vi "数字量输出配置.vi"() -> ()   [LabVIEW 2010] (continued)
            n7296 = local write "输入值_26"(w975) -> ()
            n7297 = local write "输入值_27"(w975) -> ()
            n7298 = local write "输入值_28"(w975) -> ()
            n7299 = local write "输入值_29"(w975) -> ()
            n7300 = local write "输入值_30"(w975) -> ()
            n7301 = local write "输入值_31"(w975) -> ()
            n7302 = local write "输入值_32"(w975) -> ()
            n7303 = local write "输入值_33"(w975) -> ()
            n7304 = local write "输入值_34"(w975) -> ()
            n7305 = local write "输入值_35"(w975) -> ()
            n7306 = local write "输入值_36"(w975) -> ()
            n7307 = local write "输入值_37"(w975) -> ()
            n7308 = local write "输入值_38"(w975) -> ()
            n7309 = local write "输入值_39"(w975) -> ()
            n7310 = local write "输入值_40"(w975) -> ()
            n7311 = local write "输入值_41"(w975) -> ()
            n7312 = local write "输入值_42"(w975) -> ()
            n7313 = local write "输入值_43"(w975) -> ()
            n7314 = local write "输入值_44"(w975) -> ()
            n7315 = local write "输入值_45"(w975) -> ()
            n7316 = local write "输入值_46"(w975) -> ()
            n7317 = local write "输入值_47"(w975) -> ()
            n7318 = local write "输入值_48"(w975) -> ()
            n7319 = local write "输入值_49"(w975) -> ()
            n7320 = local write "输入值_50"(w975) -> ()
            n7321 = local write "输入值_51"(w975) -> ()
            n7322 = local write "输入值_52"(w975) -> ()
            n7323 = local write "输入值_53"(w975) -> ()
            n7324 = local write "输入值_54"(w975) -> ()
            n7325 = local write "输入值_55"(w975) -> ()
            n7326 = local write "输入值_56"(w975) -> ()
            n7327 = local write "输入值_57"(w975) -> ()
            n7328 = local write "输入值_58"(w975) -> ()
            n7329 = local write "输入值_59"(w975) -> ()
            n7330 = local write "输入值_60"(w975) -> ()
            n7331 = local write "输入值_61"(w975) -> ()
            n7332 = local write "输入值_62"(w975) -> ()
            n7333 = local write "输入值_63"(w975) -> ()
            n7334 = local write "输入值_64"(w975) -> ()
            n7335 = local write "输入值_65"(w975) -> ()
            n7336 = local write "输入值_66"(w975) -> ()
            n7337 = local write "输入值_67"(w975) -> ()
            n7338 = local write "输入值_68"(w975) -> ()
            n7339 = local write "输入值_69"(w975) -> ()
            n7340 = local write "输入值_70"(w975) -> ()
            n7341 = local write "输入值_71"(w975) -> ()
            n7342 = local write "输入值_72"(w975) -> ()
            n7343 = local write "输入值_73"(w975) -> ()
            n7344 = local write "输入值_74"(w975) -> ()
            n7345 = local write "输入值_75"(w975) -> ()
            n7346 = local write "输入值_76"(w975) -> ()
            n7347 = local write "输入值_77"(w975) -> ()
            n7348 = local write "输入值_78"(w975) -> ()
            n7349 = local write "输入值_79"(w975) -> ()
            n7350 = local write "输入值_80"(w975) -> ()
          }
          event "btn_置0": Value Change {
            w976 = enum16{"0", "1"}."0" ("输入值_41")
            n7351 = event-data() -> ()  [unwired: 1 in, 5 out]
            n7352 = local write "输入值_1"(w976) -> ()
            n7353 = local write "输入值_2"(w976) -> ()
            n7354 = local write "输入值_3"(w976) -> ()
            n7355 = local write "输入值_4"(w976) -> ()
            n7356 = local write "输入值_5"(w976) -> ()
            n7357 = local write "输入值_6"(w976) -> ()
            n7358 = local write "输入值_7"(w976) -> ()
            n7359 = local write "输入值_8"(w976) -> ()
            n7360 = local write "输入值_9"(w976) -> ()
            n7361 = local write "输入值_10"(w976) -> ()
            n7362 = local write "输入值_11"(w976) -> ()
            n7363 = local write "输入值_12"(w976) -> ()
            n7364 = local write "输入值_13"(w976) -> ()
            n7365 = local write "输入值_14"(w976) -> ()
            n7366 = local write "输入值_15"(w976) -> ()
            n7367 = local write "输入值_16"(w976) -> ()
            n7368 = local write "输入值_17"(w976) -> ()
            n7369 = local write "输入值_18"(w976) -> ()
            n7370 = local write "输入值_19"(w976) -> ()
            n7371 = local write "输入值_20"(w976) -> ()
            n7372 = local write "输入值_21"(w976) -> ()
            n7373 = local write "输入值_22"(w976) -> ()
            n7374 = local write "输入值_23"(w976) -> ()
            n7375 = local write "输入值_24"(w976) -> ()
            n7376 = local write "输入值_25"(w976) -> ()
            n7377 = local write "输入值_26"(w976) -> ()
            n7378 = local write "输入值_27"(w976) -> ()
            n7379 = local write "输入值_28"(w976) -> ()
            n7380 = local write "输入值_29"(w976) -> ()
            n7381 = local write "输入值_30"(w976) -> ()
            n7382 = local write "输入值_31"(w976) -> ()
            n7383 = local write "输入值_32"(w976) -> ()
            n7384 = local write "输入值_33"(w976) -> ()
            n7385 = local write "输入值_34"(w976) -> ()
            n7386 = local write "输入值_35"(w976) -> ()
            n7387 = local write "输入值_36"(w976) -> ()
            n7388 = local write "输入值_37"(w976) -> ()
            n7389 = local write "输入值_38"(w976) -> ()
            n7390 = local write "输入值_39"(w976) -> ()
            n7391 = local write "输入值_40"(w976) -> ()
            n7392 = local write "输入值_41"(w976) -> ()
            n7393 = local write "输入值_42"(w976) -> ()
            n7394 = local write "输入值_43"(w976) -> ()
            n7395 = local write "输入值_44"(w976) -> ()
            n7396 = local write "输入值_45"(w976) -> ()
            n7397 = local write "输入值_46"(w976) -> ()
            n7398 = local write "输入值_47"(w976) -> ()
            n7399 = local write "输入值_48"(w976) -> ()
            n7400 = local write "输入值_49"(w976) -> ()
            n7401 = local write "输入值_50"(w976) -> ()
            n7402 = local write "输入值_51"(w976) -> ()
            n7403 = local write "输入值_52"(w976) -> ()
            n7404 = local write "输入值_53"(w976) -> ()
            n7405 = local write "输入值_54"(w976) -> ()
            n7406 = local write "输入值_55"(w976) -> ()
            n7407 = local write "输入值_56"(w976) -> ()
            n7408 = local write "输入值_57"(w976) -> ()
            n7409 = local write "输入值_58"(w976) -> ()
            n7410 = local write "输入值_59"(w976) -> ()
            n7411 = local write "输入值_60"(w976) -> ()
            n7412 = local write "输入值_61"(w976) -> ()
            n7413 = local write "输入值_62"(w976) -> ()
            n7414 = local write "输入值_63"(w976) -> ()
            n7415 = local write "输入值_64"(w976) -> ()
            n7416 = local write "输入值_65"(w976) -> ()
            n7417 = local write "输入值_66"(w976) -> ()
            n7418 = local write "输入值_67"(w976) -> ()
            n7419 = local write "输入值_68"(w976) -> ()
            n7420 = local write "输入值_69"(w976) -> ()
            n7421 = local write "输入值_70"(w976) -> ()
            n7422 = local write "输入值_71"(w976) -> ()
            n7423 = local write "输入值_72"(w976) -> ()
            n7424 = local write "输入值_73"(w976) -> ()
            n7425 = local write "输入值_74"(w976) -> ()
            n7426 = local write "输入值_75"(w976) -> ()
            n7427 = local write "输入值_76"(w976) -> ()
            n7428 = local write "输入值_77"(w976) -> ()
            n7429 = local write "输入值_78"(w976) -> ()
            n7430 = local write "输入值_79"(w976) -> ()
            n7431 = local write "输入值_80"(w976) -> ()
          }
        }
      }
      n7432 = Obtain Notifier(name (unnamed)=w188, notification data type=w188) -> (notifier out=w190:refnum<notifier>, error out=w189:errorcluster)  [unwired: 2 in, 1 out]
      n7433 = while {
        tunnel: w190 -> [w477]
        tunnel: w189 -> [w476]
        tunnel: [w475] -> w187
        tunnel: [w474] -> w186
        stop <- w478 stop-if-true
        n7434 = Wait Until Next ms Multiple(millisecond multiple=u32 20 ("毫秒倍数")) -> ()  [unwired: 1 out]
        n7435 = Wait on Notification(notifier=w477, timeout in ms (-1)=20 ("超时毫秒(-1)"), error in (no error)=w476) -> (notifier out=w475:refnum<notifier>, notification=w483:string, error out=w474:errorcluster)  [unwired: 1 in, 1 out]
        n7436 = Equal?(x=w483, y="DOutput" ("通知")) -> (x = y?=w481:bool)
        n7437 = case shown="真" w481 {
          frame False {
          }
          frame True {
            n7438 = while {
              stop <- w485 stop-if-true
              n7439 = local read "保持输出"() -> (w484:bool)
              n7440 = case shown="真" w484 {
                selector: w484 -> [_ w519]
                tunnel: [w490 w520] -> w487
                tunnel: [w489 w518] -> w486
                frame False {
                  n7441 = stacked-sequence {
                    tunnel: [_ w514] -> w489
                    tunnel: [w492 _] -> w490
                    frame #0 {
                      n7442 = local read "同步_A2"() -> (w494:i32)
                      n7443 = local read "同步_A1"() -> (w491:i32)
                      n7444 = Equal?(x=w491, y=w494) -> (x = y?=w493:bool)
                      n7445 = case shown="真" w493 {
                        tunnel: [FALSE w496] -> w492
                        frame False {
                        }
                        frame True {
                          n7446 = stacked-sequence {
                            tunnel: [_ w506 _] -> w496
                            frame #0 {
                              w498 = "DOCheckStart" ("名称（未命名）")
                              n7447 = Obtain Notifier(name (unnamed)=w498, notification data type=w498) -> (notifier out=w499:refnum<notifier>)  [unwired: 2 in, 2 out]
                              n7448 = Send Notification(notification="DOCheck" ("通知"), notifier=w499) -> ()  [unwired: 1 in, 2 out]
                            }
                            frame #1 {
                              # "32+16+PWM+16(I/O)\n4X3=12   每次一组"
                              # "以太网发送修改数字量输出参数命令"
                              n7449 = local read "数组_输入值"() -> (w508:enum16{"0", "1"}[][])
                              n7450 = local read "同步_A1"() -> (w504:i32)
                              n7451 = call "数值转换为U16.vi"("数值数组输入"=w508) -> ("U16输出"=w505:u16[])  [unwired: 10 in]
                              n7452 = Multiply(x=w504, y=3) -> (x*y=w502:i32)
                              n7453 = Array Subset(array=w505, index=w502, length=3 ("长度")) -> (w500:u16[])
                              n7454 = call "UDP发送.vi"("发送数据"=w500, "数据区字长"=u16 3, "报文类型"=u16 1285, "发送方标识"=u16 5397) -> ("Error"=w507:cluster{"错误？":bool, "数值":i32, "字符串":string})  [unwired: 6 in]
                              n7455 = Unbundle By Name(w507) -> ("错误？"=w506:bool)
                            }
                            frame #2 {
                              n7456 = local read "同步_A1"() -> (w512:i32)
                              n7457 = Increment(x=w512) -> (x+1=w513:i32)
                              n7458 = local write "同步_A1"(w513) -> ()
                            }
                          }
                        }
                      }
                    }
                    frame #1 {
                      n7459 = local read "同步_A1"() -> (w515:i32)
                      n7460 = Equal?(x=w515, y=5) -> (x = y?=w514:bool)
                      n7461 = case shown="真" w514 {
                        frame False {
                        }
                        frame True {
                          n7462 = property on="保持输出" class="Bool (严格)"("DisabledEnum"=T1."Enabled" ("禁用")) -> ()  [unwired: 2 in, 2 out]
                        }
                      }
                    }
                  }
                }
                frame True {
                  n7463 = Not(x=w519) -> (.not. x?=w518:bool)
                  n7464 = stacked-sequence {
                    tunnel: [_ w530] -> w520
                    frame #0 {
                      w522 = "DOCheckStart" ("名称（未命名）")
                      n7465 = Obtain Notifier(name (unnamed)=w522, notification data type=w522) -> (notifier out=w523:refnum<notifier>)  [unwired: 2 in, 2 out]
                      n7466 = Send Notification(notification="DOCheck" ("通知"), notifier=w523) -> ()  [unwired: 1 in, 2 out]
                    }
                    frame #1 {
                      # "32+16+PWM+16(I/O)\n4X3=12，每次一组"
                      # "以太网发送修改数字量输出参数命令"
                      n7467 = local read "数组_输入值"() -> (w532:enum16{"0", "1"}[][])
                      n7468 = local read "同步_A1"() -> (w528:i32)
                      n7469 = call "数值转换为U16.vi"("数值数组输入"=w532) -> ("U16输出"=w529:u16[])  [unwired: 10 in]
                      n7470 = Multiply(x=w528, y=3) -> (x*y=w526:i32)
                      n7471 = Array Subset(array=w529, index=w526, length=3 ("长度")) -> (w524:u16[])
                      n7472 = call "UDP发送.vi"("发送数据"=w524, "数据区字长"=u16 3, "报文类型"=u16 1285, "发送方标识"=u16 5397) -> ("Error"=w531:cluster{"错误？":bool, "数值":i32, "字符串":string})  [unwired: 6 in]
                      n7473 = Unbundle By Name(w531) -> ("错误？"=w530:bool)
                    }
                  }
                }
              }
              n7474 = Wait Until Next ms Multiple(millisecond multiple=u32 25 ("毫秒倍数")) -> ()  [unwired: 1 out]
              n7475 = Or(x=w487, y=w486) -> (x .or. y?=w485:bool)
            }
          }
        }
        n7476 = local read "关闭？"() -> (w478:bool)
      }
      n7477 = Release Notifier(notifier=w187, error in (no error)=w186) -> ()  [unwired: 1 in, 3 out]
      n7478 = Obtain Notifier(name (unnamed)=w185, notification data type=w185) -> (notifier out=w184:refnum<notifier>, error out=w183:errorcluster)  [unwired: 2 in, 1 out]
      n7479 = while {
        tunnel: w184 -> [w194]
        tunnel: w183 -> [w193]
        tunnel: [w192] -> w182
        tunnel: [w191] -> w181
        stop <- w196 stop-if-true
        n7480 = Wait Until Next ms Multiple(millisecond multiple=u32 20 ("毫秒倍数")) -> ()  [unwired: 1 out]
        n7481 = Wait on Notification(notifier=w194, timeout in ms (-1)=20 ("超时毫秒(-1)"), error in (no error)=w193) -> (notifier out=w192:refnum<notifier>, notification=w197:string, error out=w191:errorcluster)  [unwired: 1 in, 1 out]
        n7482 = Equal?(x=w197, y="DOCheck" ("通知")) -> (x = y?=w195:bool)
        n7483 = case shown="真" w195 {
          frame False {
          }
          frame True {
            n7484 = stacked-sequence {
              frame #0 {
                w203 = u16 0
                w207 = u16 5397
                # "异常"
                # "正常"
                n7485 = Build Array(w207, u16 1285, w203) -> (w209:u16[])
                n7486 = Build Array(w207, u16 34181, u16 0 ("元素")) -> (w206:u16[])
                n7487 = Add(x=w203, y=u16 4) -> (x+y=w201:u16)
                n7488 = call "UDP接收.vi"("匹配帧信息_异常"=w206, "长度"=w201, "匹配帧信息_正常"=w209) -> ("异常_找到?"=w212:bool, "接收超时?"=w211:bool, "正常_找到?"=w204:bool)  [unwired: 5 in, 1 out]
                n7489 = case shown="真" w204 {
                  frame False {
                    n7490 = disable-structure shown="禁用" {
                      frame Disabled {
                        n7491 = call "显示对话框信息4"("Message"="以太网接收数据错误") -> ()  [unwired: 9 in, 2 out]
                      }
                      frame Enabled {
                      }
                    }
                  }
                  frame True {
                    n7492 = local read "保持输出"() -> (w223:bool)
                    n7493 = local read "数组_输入值"() -> (w227:enum16{"0", "1"}[][])
                    n7494 = local read "数组_选择?"() -> (w228:bool[][])
                    n7495 = local read "CAN端口"() -> (w229:u16)
                    n7496 = case shown="假" w223 {
                      tunnel: [w231 w232] -> w226
                      frame False {
                        n7497 = local read "同步_A2"() -> (w231:i32)
                      }
                      frame True {
                        n7498 = local read "同步_A1"() -> (w232:i32)
                      }
                    }
                    n7499 = Index Array(array=w228, index (row)=w226) -> (element=w224:bool[])  [unwired: 1 in]
                    n7500 = To Unsigned Byte Integer(number=w226) -> (unsigned 8bit integer=w222:u8)
                    n7501 = Index Array(array=w227, index (row)=w226) -> (element=w230:enum16{"0", "1"}[])  [unwired: 1 in]
                    n7502 = Or Array Elements(Boolean array=w224) -> (logical OR=w225:bool)
                    n7503 = case shown="真" w225 {
                      tunnel: w230 -> [_ w234]
                      tunnel: w222 -> [_ w238]
                      tunnel: w229 -> [_ w237]
                      tunnel: w226 -> [_ w236]
                      tunnel: w224 -> [_ w235]
                      frame False {
                      }
                      frame True {
                        n7504 = call "16路数字量输出.vi"("第几组数据"=w238, "CAN端口"=w237) -> ("成功?"=w233:bool)  [unwired: 9 in]
                        n7505 = case shown="真" w233 {
                          tunnel: w236 -> [_ w261]
                          tunnel: w235 -> [_ w253]
                          tunnel: w234 -> [_ w251]
                          frame False {
                          }
                          frame True {
                            n7506 = call "DAQNavi Assistant2"() -> ("dataOut(U8Array)"=w249:u8[])  [unwired: 2 in, 17 out]
                            n7507 = Index Array(array=w249, index #1=0 ("索引"), index #2=1 ("索引")) -> (element #1=w246:u8, element #2=w245:u8)
                            n7508 = local read "保持输出"() -> (w239:bool)
                            n7509 = Number To Boolean Array(number=w246) -> (Boolean array=w242:bool[])
                            n7510 = Number To Boolean Array(number=w245) -> (Boolean array=w241:bool[])
                            n7511 = Build Array (concatenate)(w242, w241) -> (w244:bool[])
                            n7512 = Boolean To (0,1)(Boolean=w244) -> (0, 1=w243:i16[])
                            n7513 = case shown="真" w239 {
                              tunnel: [w262 w263] -> w240
                              frame False {
                                n7514 = local read "同步_A2"() -> (w262:i32)
                              }
                              frame True {
                                n7515 = local read "同步_A1"() -> (w263:i32)
                              }
                            }
                            n7516 = for {
                              tunnel: w243 -> [w269] mode=indexing
                              tunnel: w251 -> [w268] mode=indexing
                              tunnel: w253 -> [w267] mode=indexing
                              tunnel: [w264] -> w254 mode=indexing
                              tunnel: [w265] -> w255 mode=indexing
                              tunnel: [w266] -> w250 mode=indexing
                              n7517 = case shown="真" w267 {
                                tunnel: w269 -> [_ w277]
                                tunnel: w268 -> [_ w279]
                                tunnel: [cluster{u32, u32}[] [{12369084, 12369084}] ("结果") w273] -> w264
                                tunnel: ["" w275] -> w265
                                tunnel: [TRUE w274] -> w266
                                frame False {
                                }
                                frame True {
                                n7518 = To Word Integer(number=w279) -> (16bit integer=w278:i16)
                                n7519 = Equal To 0?(x=w277) -> (x = 0?=w276:bool)
                                n7520 = Equal?(x=w277, y=w278) -> (x = y?=w274:bool)
                                n7521 = case shown="假" w274 {
                                tunnel: [cluster{u32, u32}[] [{16711680, 16711680}] ("结果") cluster{u32, u32}[] [{6618880, 6618880}] ("结果")] -> w273
                                frame False {
                                }
                                frame True {
                                }
                                }
                                n7522 = case shown="真" w276 {
                                tunnel: ["1" "0"] -> w275
                                frame False {
                                }
                                frame True {
                                }
                                }
                                }
                              }
                            }
                            n7523 = local read "测试结论"() -> (w259:string)
                            n7524 = And Array Elements(Boolean array=w250) -> (logical AND=w252:bool)
                            n7525 = case shown="真" w252 {
                              tunnel: ["被测板卡所选择的数字量输出%d组测试故障，具体见上面试验结论！" "被测板卡所选择的数字量输出%d组测试正常！"] -> w257
                              frame False {
                              }
                              frame True {
                              }
                            }
                            n7526 = Format Into String(format string=w257, w240) -> (resulting string=w260:string)  [unwired: 2 in, 1 out]
                            n7527 = Concatenate Strings(w259, w260, "\r") -> (w256:string)
                            n7528 = local write "测试结论"(w256) -> ()
                            n7529 = case shown="4" w261 {
                              tunnel: w254 -> [w288 w341 w378 w415 w452]
                              tunnel: w255 -> [w284 w322 w359 w395 w432]
                              frame 0, Default {
                                n7530 = local read "D_IN_1"() -> (w287:string[][])
                                n7531 = Replace Array Subset(array=w287, new element=w284, index (col)=2 ("禁用的索引 (列)")) -> (w285:string[][])  [unwired: 1 in]
                                n7532 = Index Array(array=w288, index (row) #1=0 ("索引"), index (row) #2=1 ("索引"), index (row) #3=2 ("索引"), index (row) #4=3 ("索引"), index (row) #5=4 ("索引"), index (row) #6=5 ("索引"), index (row) #7=6 ("索引"), index (row) #8=7 ("索引"), index (row) #9=8 ("索引"), index (row) #10=9 ("索引"), index (row) #11=10 ("索引"), index (row) #12=11 ("索引"), index (row) #13=12 ("索引"), index (row) #14=13 ("索引"), index (row) #15=14 ("索引"), index (row) #16=15 ("索引")) -> (element #1=w304:cluster{u32, u32}[], element #2=w303:cluster{u32, u32}[], element #3=w302:cluster{u32, u32}[], element #4=w301:cluster{u32, u32}[], element #5=w300:cluster{u32, u32}[], element #6=w289:cluster{u32, u32}[], element #7=w290:cluster{u32, u32}[], element #8=w291:cluster{u32, u32}[], element #9=w292:cluster{u32, u32}[], element #10=w293:cluster{u32, u32}[], element #11=w294:cluster{u32, u32}[], element #12=w295:cluster{u32, u32}[], element #13=w296:cluster{u32, u32}[], element #14=w297:cluster{u32, u32}[], element #15=w298:cluster{u32, u32}[], element #16=w299:cluster{u32, u32}[])  [unwired: 16 in]
                                n7533 = local write "D_IN_1"(w285) -> ()
                                n7534 = property on="light_1" class="Bool (严格)"("Colors [4]"=w304) -> ()  [unwired: 2 in, 2 out]
                                n7535 = property on="light_2" class="Bool (严格)"("Colors [4]"=w303) -> ()  [unwired: 2 in, 2 out]
                                n7536 = property on="light_3" class="Bool (严格)"("Colors [4]"=w302) -> ()  [unwired: 2 in, 2 out]
                                n7537 = property on="light_4" class="Bool (严格)"("Colors [4]"=w301) -> ()  [unwired: 2 in, 2 out]
                                n7538 = property on="light_5" class="Bool (严格)"("Colors [4]"=w300) -> ()  [unwired: 2 in, 2 out]
                                n7539 = property on="light_6" class="Bool (严格)"("Colors [4]"=w289) -> ()  [unwired: 2 in, 2 out]
                                n7540 = property on="light_7" class="Bool (严格)"("Colors [4]"=w290) -> ()  [unwired: 2 in, 2 out]
                                n7541 = property on="light_8" class="Bool (严格)"("Colors [4]"=w291) -> ()  [unwired: 2 in, 2 out]
                                n7542 = property on="light_9" class="Bool (严格)"("Colors [4]"=w292) -> ()  [unwired: 2 in, 2 out]
                                n7543 = property on="light_10" class="Bool (严格)"("Colors [4]"=w293) -> ()  [unwired: 2 in, 2 out]
                                n7544 = property on="light_11" class="Bool (严格)"("Colors [4]"=w294) -> ()  [unwired: 2 in, 2 out]
                                n7545 = property on="light_12" class="Bool (严格)"("Colors [4]"=w295) -> ()  [unwired: 2 in, 2 out]
                                n7546 = property on="light_13" class="Bool (严格)"("Colors [4]"=w296) -> ()  [unwired: 2 in, 2 out]
                                n7547 = property on="light_14" class="Bool (严格)"("Colors [4]"=w297) -> ()  [unwired: 2 in, 2 out]
                                n7548 = property on="light_15" class="Bool (严格)"("Colors [4]"=w298) -> ()  [unwired: 2 in, 2 out]
                                n7549 = property on="light_16" class="Bool (严格)"("Colors [4]"=w299) -> ()  [unwired: 2 in, 2 out]
                              }
                              frame 2 {
                                n7550 = local read "D_IN_3"() -> (w323:string[][])
                                n7551 = Replace Array Subset(array=w323, new element=w322, index (col)=2 ("索引 (列)")) -> (w321:string[][])  [unwired: 1 in]
                                n7552 = Index Array(array=w341, index (row) #1=0 ("索引"), index (row) #2=1 ("索引"), index (row) #3=2 ("索引"), index (row) #4=3 ("索引"), index (row) #5=4 ("索引"), index (row) #6=5 ("索引"), index (row) #7=6 ("索引"), index (row) #8=7 ("索引"), index (row) #9=8 ("索引"), index (row) #10=9 ("索引"), index (row) #11=10 ("索引"), index (row) #12=11 ("索引"), index (row) #13=12 ("索引"), index (row) #14=13 ("索引"), index (row) #15=14 ("索引"), index (row) #16=15 ("索引")) -> (element #1=w340:cluster{u32, u32}[], element #2=w339:cluster{u32, u32}[], element #3=w338:cluster{u32, u32}[], element #4=w337:cluster{u32, u32}[], element #5=w336:cluster{u32, u32}[], element #6=w335:cluster{u32, u32}[], element #7=w334:cluster{u32, u32}[], element #8=w333:cluster{u32, u32}[], element #9=w332:cluster{u32, u32}[], element #10=w331:cluster{u32, u32}[], element #11=w330:cluster{u32, u32}[], element #12=w329:cluster{u32, u32}[], element #13=w328:cluster{u32, u32}[], element #14=w327:cluster{u32, u32}[], element #15=w326:cluster{u32, u32}[], element #16=w325:cluster{u32, u32}[])  [unwired: 16 in]
                                n7553 = local write "D_IN_3"(w321) -> ()
                                n7554 = property on="light_33" class="Bool (严格)"("Colors [4]"=w340) -> ()  [unwired: 2 in, 2 out]
                                n7555 = property on="light_34" class="Bool (严格)"("Colors [4]"=w339) -> ()  [unwired: 2 in, 2 out]
                                n7556 = property on="light_35" class="Bool (严格)"("Colors [4]"=w338) -> ()  [unwired: 2 in, 2 out]
                                n7557 = property on="light_36" class="Bool (严格)"("Colors [4]"=w337) -> ()  [unwired: 2 in, 2 out]
                                n7558 = property on="light_37" class="Bool (严格)"("Colors [4]"=w336) -> ()  [unwired: 2 in, 2 out]
                                n7559 = property on="light_38" class="Bool (严格)"("Colors [4]"=w335) -> ()  [unwired: 2 in, 2 out]
                                n7560 = property on="light_39" class="Bool (严格)"("Colors [4]"=w334) -> ()  [unwired: 2 in, 2 out]
                                n7561 = property on="light_40" class="Bool (严格)"("Colors [4]"=w333) -> ()  [unwired: 2 in, 2 out]
                                n7562 = property on="light_41" class="Bool (严格)"("Colors [4]"=w332) -> ()  [unwired: 2 in, 2 out]
                                n7563 = property on="light_42" class="Bool (严格)"("Colors [4]"=w331) -> ()  [unwired: 2 in, 2 out]
                                n7564 = property on="light_43" class="Bool (严格)"("Colors [4]"=w330) -> ()  [unwired: 2 in, 2 out]
                                n7565 = property on="light_44" class="Bool (严格)"("Colors [4]"=w329) -> ()  [unwired: 2 in, 2 out]
                                n7566 = property on="light_45" class="Bool (严格)"("Colors [4]"=w328) -> ()  [unwired: 2 in, 2 out]
                                n7567 = property on="light_46" class="Bool (严格)"("Colors [4]"=w327) -> ()  [unwired: 2 in, 2 out]
                                n7568 = property on="light_47" class="Bool (严格)"("Colors [4]"=w326) -> ()  [unwired: 2 in, 2 out]
                                n7569 = property on="light_48" class="Bool (严格)"("Colors [4]"=w325) -> ()  [unwired: 2 in, 2 out]
                              }
                              frame 3 {
                                n7570 = local read "D_IN_4"() -> (w360:string[][])
                                n7571 = Replace Array Subset(array=w360, new element=w359, index (col)=2 ("索引 (列)")) -> (w358:string[][])  [unwired: 1 in]
                                n7572 = Index Array(array=w378, index (row) #1=0 ("索引"), index (row) #2=1 ("索引"), index (row) #3=2 ("索引"), index (row) #4=3 ("索引"), index (row) #5=4 ("索引"), index (row) #6=5 ("索引"), index (row) #7=6 ("索引"), index (row) #8=7 ("索引"), index (row) #9=8 ("索引"), index (row) #10=9 ("索引"), index (row) #11=10 ("索引"), index (row) #12=11 ("索引"), index (row) #13=12 ("索引"), index (row) #14=13 ("索引"), index (row) #15=14 ("索引"), index (row) #16=15 ("索引")) -> (element #1=w377:cluster{u32, u32}[], element #2=w376:cluster{u32, u32}[], element #3=w375:cluster{u32, u32}[], element #4=w374:cluster{u32, u32}[], element #5=w373:cluster{u32, u32}[], element #6=w372:cluster{u32, u32}[], element #7=w371:cluster{u32, u32}[], element #8=w370:cluster{u32, u32}[], element #9=w369:cluster{u32, u32}[], element #10=w368:cluster{u32, u32}[], element #11=w367:cluster{u32, u32}[], element #12=w366:cluster{u32, u32}[], element #13=w365:cluster{u32, u32}[], element #14=w364:cluster{u32, u32}[], element #15=w363:cluster{u32, u32}[], element #16=w362:cluster{u32, u32}[])  [unwired: 16 in]
                                n7573 = local write "D_IN_4"(w358) -> ()
                                n7574 = property on="light_49" class="Bool (严格)"("Colors [4]"=w377) -> ()  [unwired: 2 in, 2 out]
                                n7575 = property on="light_50" class="Bool (严格)"("Colors [4]"=w376) -> ()  [unwired: 2 in, 2 out]
                                n7576 = property on="light_51" class="Bool (严格)"("Colors [4]"=w375) -> ()  [unwired: 2 in, 2 out]
                                n7577 = property on="light_52" class="Bool (严格)"("Colors [4]"=w374) -> ()  [unwired: 2 in, 2 out]
                                n7578 = property on="light_53" class="Bool (严格)"("Colors [4]"=w373) -> ()  [unwired: 2 in, 2 out]
                                n7579 = property on="light_54" class="Bool (严格)"("Colors [4]"=w372) -> ()  [unwired: 2 in, 2 out]
                                n7580 = property on="light_55" class="Bool (严格)"("Colors [4]"=w371) -> ()  [unwired: 2 in, 2 out]
                                n7581 = property on="light_56" class="Bool (严格)"("Colors [4]"=w370) -> ()  [unwired: 2 in, 2 out]
                                n7582 = property on="light_57" class="Bool (严格)"("Colors [4]"=w369) -> ()  [unwired: 2 in, 2 out]
                                n7583 = property on="light_58" class="Bool (严格)"("Colors [4]"=w368) -> ()  [unwired: 2 in, 2 out]
                                n7584 = property on="light_59" class="Bool (严格)"("Colors [4]"=w367) -> ()  [unwired: 2 in, 2 out]
                                n7585 = property on="light_60" class="Bool (严格)"("Colors [4]"=w366) -> ()  [unwired: 2 in, 2 out]
                                n7586 = property on="light_61" class="Bool (严格)"("Colors [4]"=w365) -> ()  [unwired: 2 in, 2 out]
                                n7587 = property on="light_62" class="Bool (严格)"("Colors [4]"=w364) -> ()  [unwired: 2 in, 2 out]
                                n7588 = property on="light_63" class="Bool (严格)"("Colors [4]"=w363) -> ()  [unwired: 2 in, 2 out]
                                n7589 = property on="light_64" class="Bool (严格)"("Colors [4]"=w362) -> ()  [unwired: 2 in, 2 out]
                              }
                              frame 4 {
                                n7590 = local read "D_IN_5"() -> (w397:string[][])
                                n7591 = Replace Array Subset(array=w397, new element=w395, index (col)=2 ("索引 (列)")) -> (w396:string[][])  [unwired: 1 in]
                                n7592 = Index Array(array=w415, index (row) #1=0 ("索引"), index (row) #2=1 ("索引"), index (row) #3=2 ("索引"), index (row) #4=3 ("索引"), index (row) #5=4 ("索引"), index (row) #6=5 ("索引"), index (row) #7=6 ("索引"), index (row) #8=7 ("索引"), index (row) #9=8 ("索引"), index (row) #10=9 ("索引"), index (row) #11=10 ("索引"), index (row) #12=11 ("索引"), index (row) #13=12 ("索引"), index (row) #14=13 ("索引"), index (row) #15=14 ("索引"), index (row) #16=15 ("索引")) -> (element #1=w414:cluster{u32, u32}[], element #2=w413:cluster{u32, u32}[], element #3=w412:cluster{u32, u32}[], element #4=w411:cluster{u32, u32}[], element #5=w410:cluster{u32, u32}[], element #6=w409:cluster{u32, u32}[], element #7=w408:cluster{u32, u32}[], element #8=w407:cluster{u32, u32}[], element #9=w406:cluster{u32, u32}[], element #10=w405:cluster{u32, u32}[], element #11=w404:cluster{u32, u32}[], element #12=w403:cluster{u32, u32}[], element #13=w402:cluster{u32, u32}[], element #14=w401:cluster{u32, u32}[], element #15=w400:cluster{u32, u32}[], element #16=w399:cluster{u32, u32}[])  [unwired: 16 in]
                                n7593 = local write "D_IN_5"(w396) -> ()
                                n7594 = property on="light_65" class="Bool (严格)"("Colors [4]"=w414) -> ()  [unwired: 2 in, 2 out]
                                n7595 = property on="light_66" class="Bool (严格)"("Colors [4]"=w413) -> ()  [unwired: 2 in, 2 out]
                                n7596 = property on="light_67" class="Bool (严格)"("Colors [4]"=w412) -> ()  [unwired: 2 in, 2 out]
                                n7597 = property on="light_68" class="Bool (严格)"("Colors [4]"=w411) -> ()  [unwired: 2 in, 2 out]
                                n7598 = property on="light_69" class="Bool (严格)"("Colors [4]"=w410) -> ()  [unwired: 2 in, 2 out]
                                n7599 = property on="light_70" class="Bool (严格)"("Colors [4]"=w409) -> ()  [unwired: 2 in, 2 out]
                                n7600 = property on="light_71" class="Bool (严格)"("Colors [4]"=w408) -> ()  [unwired: 2 in, 2 out]
                                n7601 = property on="light_72" class="Bool (严格)"("Colors [4]"=w407) -> ()  [unwired: 2 in, 2 out]
                                n7602 = property on="light_73" class="Bool (严格)"("Colors [4]"=w406) -> ()  [unwired: 2 in, 2 out]
                                n7603 = property on="light_74" class="Bool (严格)"("Colors [4]"=w405) -> ()  [unwired: 2 in, 2 out]
                                n7604 = property on="light_75" class="Bool (严格)"("Colors [4]"=w404) -> ()  [unwired: 2 in, 2 out]
                                n7605 = property on="light_76" class="Bool (严格)"("Colors [4]"=w403) -> ()  [unwired: 2 in, 2 out]
                                n7606 = property on="light_77" class="Bool (严格)"("Colors [4]"=w402) -> ()  [unwired: 2 in, 2 out]
                                n7607 = property on="light_78" class="Bool (严格)"("Colors [4]"=w401) -> ()  [unwired: 2 in, 2 out]
                                n7608 = property on="light_79" class="Bool (严格)"("Colors [4]"=w400) -> ()  [unwired: 2 in, 2 out]
                                n7609 = property on="light_80" class="Bool (严格)"("Colors [4]"=w399) -> ()  [unwired: 2 in, 2 out]
                              }
                              frame 1 {
                                n7610 = local read "D_IN_2"() -> (w434:string[][])
                                n7611 = Replace Array Subset(array=w434, new element=w432, index (col)=2 ("索引 (列)")) -> (w433:string[][])  [unwired: 1 in]
                                n7612 = Index Array(array=w452, index (row) #1=0 ("索引"), index (row) #2=1 ("索引"), index (row) #3=2 ("索引"), index (row) #4=3 ("索引"), index (row) #5=4 ("索引"), index (row) #6=5 ("索引"), index (row) #7=6 ("索引"), index (row) #8=7 ("索引"), index (row) #9=8 ("索引"), index (row) #10=9 ("索引"), index (row) #11=10 ("索引"), index (row) #12=11 ("索引"), index (row) #13=12 ("索引"), index (row) #14=13 ("索引"), index (row) #15=14 ("索引"), index (row) #16=15 ("索引")) -> (element #1=w451:cluster{u32, u32}[], element #2=w450:cluster{u32, u32}[], element #3=w449:cluster{u32, u32}[], element #4=w448:cluster{u32, u32}[], element #5=w447:cluster{u32, u32}[], element #6=w446:cluster{u32, u32}[], element #7=w445:cluster{u32, u32}[], element #8=w444:cluster{u32, u32}[], element #9=w443:cluster{u32, u32}[], element #10=w442:cluster{u32, u32}[], element #11=w441:cluster{u32, u32}[], element #12=w440:cluster{u32, u32}[], element #13=w439:cluster{u32, u32}[], element #14=w438:cluster{u32, u32}[], element #15=w437:cluster{u32, u32}[], element #16=w436:cluster{u32, u32}[])  [unwired: 16 in]
                                n7613 = local write "D_IN_2"(w433) -> ()
                                n7614 = property on="light_17" class="Bool (严格)"("Colors [4]"=w451) -> ()  [unwired: 2 in, 2 out]
                                n7615 = property on="light_18" class="Bool (严格)"("Colors [4]"=w450) -> ()  [unwired: 2 in, 2 out]
                                n7616 = property on="light_19" class="Bool (严格)"("Colors [4]"=w449) -> ()  [unwired: 2 in, 2 out]
                                n7617 = property on="light_20" class="Bool (严格)"("Colors [4]"=w448) -> ()  [unwired: 2 in, 2 out]
                                n7618 = property on="light_21" class="Bool (严格)"("Colors [4]"=w447) -> ()  [unwired: 2 in, 2 out]
                                n7619 = property on="light_22" class="Bool (严格)"("Colors [4]"=w446) -> ()  [unwired: 2 in, 2 out]
                                n7620 = property on="light_23" class="Bool (严格)"("Colors [4]"=w445) -> ()  [unwired: 2 in, 2 out]
                                n7621 = property on="light_24" class="Bool (严格)"("Colors [4]"=w444) -> ()  [unwired: 2 in, 2 out]
                                n7622 = property on="light_25" class="Bool (严格)"("Colors [4]"=w443) -> ()  [unwired: 2 in, 2 out]
                                n7623 = property on="light_26" class="Bool (严格)"("Colors [4]"=w442) -> ()  [unwired: 2 in, 2 out]
                                n7624 = property on="light_27" class="Bool (严格)"("Colors [4]"=w441) -> ()  [unwired: 2 in, 2 out]
                                n7625 = property on="light_28" class="Bool (严格)"("Colors [4]"=w440) -> ()  [unwired: 2 in, 2 out]
                                n7626 = property on="light_29" class="Bool (严格)"("Colors [4]"=w439) -> ()  [unwired: 2 in, 2 out]
                                n7627 = property on="light_30" class="Bool (严格)"("Colors [4]"=w438) -> ()  [unwired: 2 in, 2 out]
                                n7628 = property on="light_31" class="Bool (严格)"("Colors [4]"=w437) -> ()  [unwired: 2 in, 2 out]
                                n7629 = property on="light_32" class="Bool (严格)"("Colors [4]"=w436) -> ()  [unwired: 2 in, 2 out]
                              }
                            }
                          }
                        }
                      }
                    }
                  }
                }
                n7630 = case shown="真" w211 {
                  frame False {
                  }
                  frame True {
                    n7631 = call "显示对话框信息3"("Message"="数字量输出数值修改超时") -> ("结束"=w213:bool)  [unwired: 9 in, 1 out]
                    n7632 = case shown="真" w213 {
                      frame False {
                      }
                      frame True {
                        n7633 = local write "同步_A1"(5 ("同步_A1")) -> ()
                        n7634 = local write "保持输出"(FALSE ("保持输出")) -> ()
                      }
                    }
                  }
                }
                n7635 = case shown="真" w212 {
                  frame False {
                  }
                  frame True {
                    n7636 = call "显示对话框信息2"("Message"="数字量输出数值修改失败") -> ("结束"=w217:bool)  [unwired: 9 in, 1 out]
                    n7637 = case shown="真" w217 {
                      frame False {
                      }
                      frame True {
                        n7638 = local write "同步_A1"(5 ("同步_A1")) -> ()
                        n7639 = local write "保持输出"(FALSE ("保持输出")) -> ()
                      }
                    }
                  }
                }
              }
              frame #1 {
                n7640 = local read "保持输出"() -> (w471:bool)
                n7641 = case shown="假" w471 {
                  frame False {
                    n7642 = local read "同步_A2"() -> (w472:i32)
                    n7643 = Increment(x=w472) -> (x+1=w473:i32)
                    n7644 = local write "同步_A2"(w473) -> ()
                  }
                  frame True {
                  }
                }
              }
            }
          }
        }
        n7645 = local read "关闭？"() -> (w196:bool)
      }
      n7646 = Release Notifier(notifier=w182, error in (no error)=w181) -> ()  [unwired: 1 in, 3 out]
    }
  }
  n7647 = disable-structure shown="禁用" {
    frame Disabled {
      n7648 = for {
        N: 40 -> [_]
        i -> [w982]
        n7649 = Wait Until Next ms Multiple(millisecond multiple=u32 10 ("毫秒倍数")) -> ()  [unwired: 1 out]
        n7650 = Bundle(w982, "y"=-1) -> (w981:cluster{i32, "y":i32})  [unwired: 1 in]
        n7651 = property on="D_IN_1" class="Tbl (严格)"("Active Cell"=w981) -> (error out=w980:errorcluster)  [unwired: 2 in, 1 out]
        n7652 = property on="D_IN_1" class="Tbl (严格)"(error in=w980, "Cell BG Color"=u32 12369084) -> ()  [unwired: 1 in, 2 out]
      }
    }
    frame Enabled {
    }
  }
  n7653 = disable-structure shown="禁用" {
    frame Disabled {
      n7654 = for {
        N: 40 -> [_]
        i -> [w986]
        n7655 = for {
          N: 4 -> [_]
          tunnel: w986 -> [w994]
          i -> [w991]
          n7656 = Bundle(w994, w991) -> (w990:cluster{i32, i32})  [unwired: 1 in]
          n7657 = Quotient & Remainder(x=w994, y=2) -> (x-y*floor(x/y)=w992:i32)  [unwired: 1 out]
          n7658 = property on="D_IN_1" class="Tbl (严格)"("Active Cell"=w990) -> (error out=w988:errorcluster)  [unwired: 2 in, 1 out]
          n7659 = Equal To 0?(x=w992) -> (x = 0?=w995:bool)
          n7660 = case shown="真" w995 {
            tunnel: [u32 16448250 u32 15723488] -> w989
            frame False {
            }
            frame True {
            }
          }
          n7661 = property on="D_IN_1" class="Tbl (严格)"(error in=w988, "Cell BG Color"=w989) -> ()  [unwired: 1 in, 2 out]
        }
        n7662 = Wait Until Next ms Multiple(millisecond multiple=u32 10 ("毫秒倍数")) -> ()  [unwired: 1 out]
      }
    }
    frame Enabled {
    }
  }
